vi "Open Channel Panel.vi"(8 "error in (no error)":errorcluster, 10 "Channel Index":i32, 11 "Sequencer in":refnum<class "Sequencer.lvclass">) -> (0 "error out":errorcluster, 3 "Sequencer out":refnum<class "Sequencer.lvclass">)   [LabVIEW 2015, in "Sequencer.lvlib" / "Sequencer.lvclass"]
uses:
  Sequencer.lvclass
  Sequencer.lvclass/Sequencer.ctl
  <vilib>/ActorFramework/Message Enqueuer/Message Enqueuer.lvclass/Message Enqueuer.ctl
  <vilib>/ActorFramework/Message Enqueuer/Enqueue.vi
  <vilib>/ActorFramework/Message Priority Queue/Priority Enqueue.vi
  SequencerConfig.lvclass
  <vilib>/ActorFramework/Message Enqueuer/Message Enqueuer.lvclass
  <userlib>/_Win8uiFramework/ViewableActor Messages/Open Front Panel Msg/Open Front Panel Msg.lvclass
  SequencerInfo.lvclass
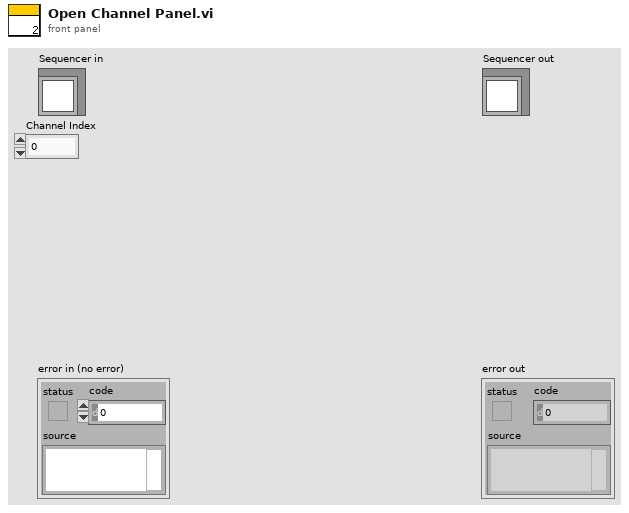
[diagram p1: front panel]
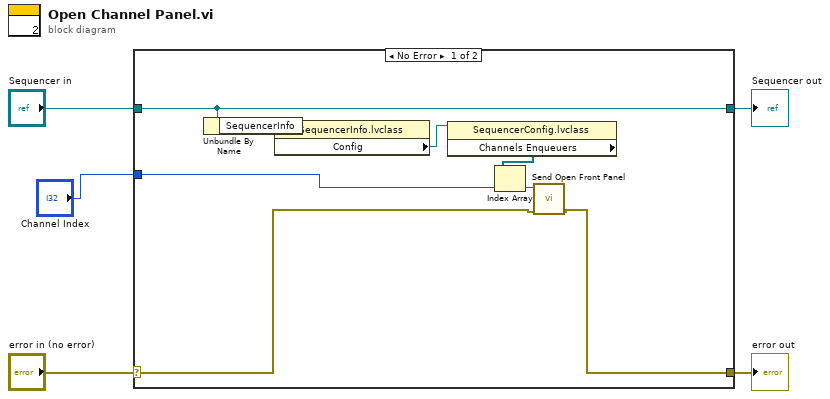
[diagram p0: block diagram]
diagram:
  n1 = case shown="No Error" "error in (no error)" {
    selector: "error in (no error)" -> [w10 w15]
    tunnel: [w11 w15] -> w4
    tunnel: [w13 w14] -> w2
    tunnel: "Sequencer in" -> [w13 w14]
    tunnel: "Channel Index" -> [w12 _]
    frame No Error {
      n2 = Unbundle By Name(w13) -> ("SequencerInfo"=w7:refnum<class "SequencerInfo.lvclass">)
      n3 = property class="SequencerInfo.lvclass"(reference=w7) -> ("Config"=w8:refnum<class "SequencerConfig.lvclass">)  [unwired: 1 in, 2 out]
      n4 = property class="SequencerConfig.lvclass"(reference=w8) -> ("Channels Enqueuers"=w6:refnum<class "Message Enqueuer.lvclass">[])  [unwired: 1 in, 2 out]
      n5 = Index Array(array=w6, index=w12) -> (element=w9:refnum<class "Message Enqueuer.lvclass">)
      n6 = call <userlib>:"Send Open Front Panel.vi"("error in (no error)"=w10, "Message Enqueuer"=w9) -> ("error out"=w11:errorcluster)  [unwired: 8 in, 1 out]
    }
    frame Error {
    }
  }
  "error out" <- w4
  "Sequencer out" <- w2
